vi "API_Get_Finite_Time.vi"(1 "Argument List":string[](array[string])) -> (0 "Finite Time":dbl)   [LabVIEW 2011]
doc: "This VI examines the given argument list and if the command is a finite mode API, it returns the value of the finite time."
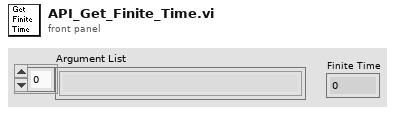
[diagram p1: front panel]
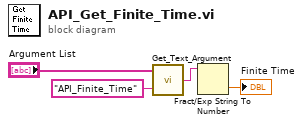
[diagram p0: block diagram]
diagram:
  n1 = call "Get_Text_Argument.vi"("Argument"="API_Finite_Time", "Argument List"="Argument List") -> ("Text"=w2:string)
  n2 = Fract/Exp String To Number(string=w2) -> (number=→"Finite Time":dbl)  [unwired: 3 in, 1 out]
